vi "Set auto start.vi"(8 "error in (no error)":errorcluster, 10 "auto start":bool, 11 "NI Digital Output in":refnum<class "NI Digital Output.lvclass">) -> (0 "error out":errorcluster, 3 "NI Digital Output out":refnum<class "NI Digital Output.lvclass">)   [LabVIEW 2020, in "NI DAQmx.lvlib" / "NI Digital Output.lvclass"]
uses:
  NI Digital Output.lvclass
  NI Digital Output.lvclass/NI Digital Output.ctl
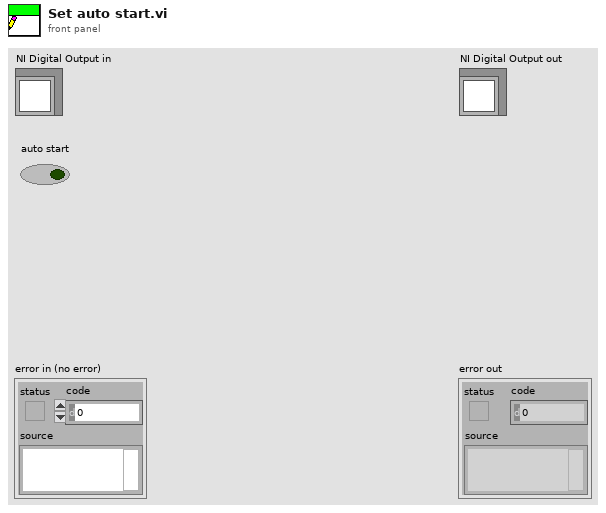
[diagram p1: front panel]
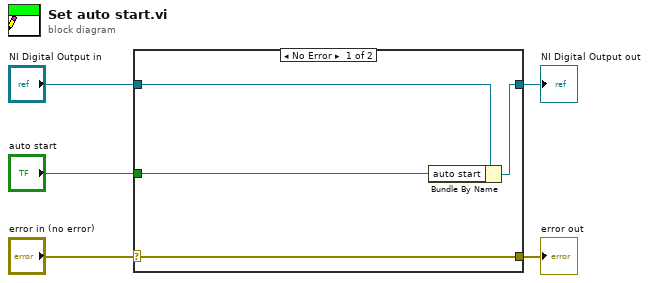
[diagram p0: block diagram]
diagram:
  n1 = case shown="No Error" "error in (no error)" {
    selector: "error in (no error)" -> [w9 w10]
    tunnel: [w9 w10] -> w4
    tunnel: [w7 w11] -> w2
    tunnel: "NI Digital Output in" -> [w8 w11]
    tunnel: "auto start" -> [w6 _]
    frame No Error {
      n2 = Bundle By Name(cluster=w8, "auto start"=w6) -> (w7:refnum<class "NI Digital Output.lvclass">)
    }
    frame Error {
    }
  }
  "error out" <- w4
  "NI Digital Output out" <- w2
